vi "Compare Strings.vi"(1 "String 2":string, 2 "String":string) -> (0 "Boolean":bool)   [LabVIEW 2025]
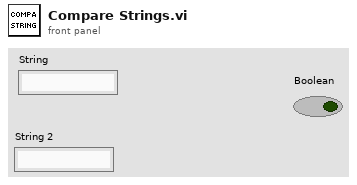
[diagram p1: front panel]
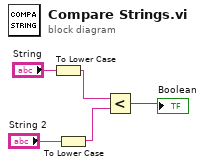
[diagram p0: block diagram]
diagram:
  n1 = To Lower Case(string="String") -> (all lower case string=w3:string)
  n2 = To Lower Case(string="String 2") -> (all lower case string=w2:string)
  n3 = Less?(x=w3, y=w2) -> (x < y?=→"Boolean":bool)
